vi "KE6221 -- Set Wave No Trig In Inactive Val.vi"(0 "Resource In":refnum<visa-resource-name>, 1 "Check For SCPI Errors? (T)":bool=TRUE, 7 "Inactive Level In (%)":T1=50.0 caption="Note:  100% = max, -100% = min" min=-100.0 max=100.0 format="%.3p", 11 "error in (no error)":errorcluster, 12 "Read Back Set Value? (T)":bool=TRUE) -> (4 "Resource Out (dupl)":refnum<visa-resource-name>, 8 "Inactive Level Out (%)":T1=50.0 caption="Note:  100% = max, -100% = min" min=-100.0 max=100.0 format="%.3p", 15 "error out":errorcluster)   [LabVIEW 2018, in "Keithley 622x.lvlib"]
uses:
  Keithley 622x.lvlib
  Typedefs/KE6221 -- Wave Inactive Level.ctl
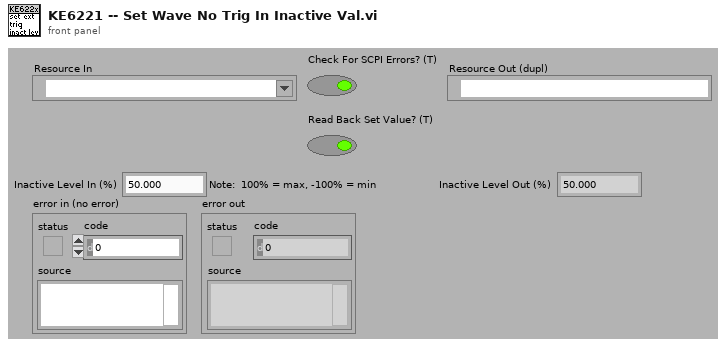
[diagram p1: front panel]
types:
  T1 = typedef "Keithley 622x.lvlib/KE6221 -- Wave Inactive Level.ctl" = dbl
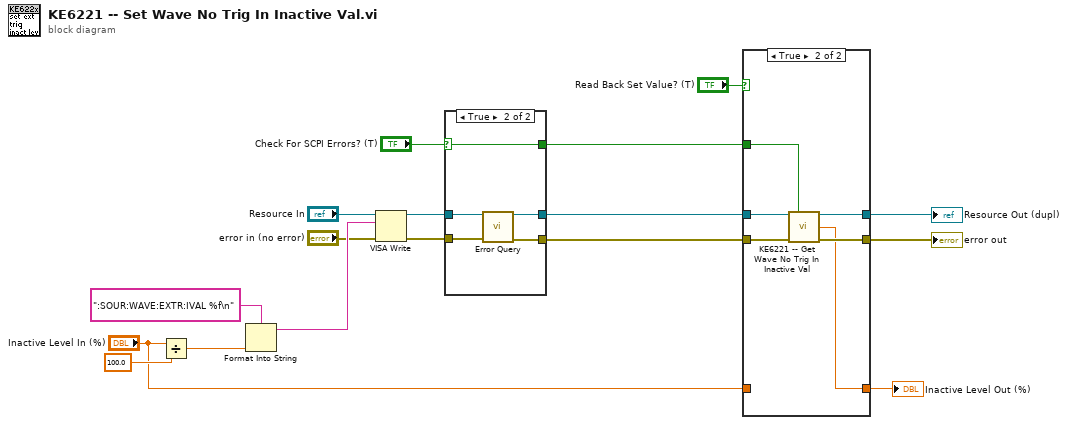
[diagram p0: block diagram]
diagram:
  n1 = Divide(x="Inactive Level In (%)", y=T1 100.0) -> (x/y=w3:T1)
  n2 = Format Into String(format string=":SOUR:WAVE:EXTR:IVAL %f\n", w3) -> (resulting string=w15:string)  [unwired: 2 in, 1 out]
  n3 = VISA Write(VISA resource name="Resource In", write buffer=w15, error in (no error)="error in (no error)") -> (VISA resource name out=w12:refnum<visa-resource-name>, error out=w11:errorcluster)  [unwired: 1 out]
  n4 = case shown="True" "Check For SCPI Errors? (T)" {
    selector: "Check For SCPI Errors? (T)" -> [w18 w21]
    tunnel: w12 -> [w20 w25]
    tunnel: w11 -> [w19 w24]
    tunnel: [w19 w23] -> w7
    tunnel: [w20 w22] -> w10
    tunnel: [w18 w21] -> w8
    frame False {
    }
    frame True {
      n5 = call "Error Query.vi"("VISA Resource In"=w25, "error in (no error)"=w24) -> ("VISA Resource Out (dupl)"=w22:refnum<visa-resource-name>, "error out"=w23:errorcluster)  [unwired: 10 in, 2 out]
    }
  }
  n6 = case shown="True" "Read Back Set Value? (T)" {
    tunnel: w10 -> [w27 w34]
    tunnel: w8 -> [_ w33]
    tunnel: w7 -> [w26 w32]
    tunnel: "Inactive Level In (%)" -> [w28 _]
    tunnel: [w28 w29] -> w1
    tunnel: [w27 w31] -> w6
    tunnel: [w26 w30] -> w5
    frame False {
    }
    frame True {
      n7 = call "KE6221 -- Get Wave No Trig In Inactive Val.vi"("Resource In"=w34, "Check For SCPI Errors? (T)"=w33, "error in (no error)"=w32) -> ("Resource Out (dupl)"=w31:refnum<visa-resource-name>, "Inactive Level (%)"=w29:T1, "error out"=w30:errorcluster)  [unwired: 10 in]
    }
  }
  "Resource Out (dupl)" <- w6
  "error out" <- w5
  "Inactive Level Out (%)" <- w1
